vi "Main.vi"() -> ()   [LabVIEW 2018]
doc: "Use this template to build a producer/consumer design pattern with events to produce queue items. Use this design pattern instead of the User Interface Event Handler pattern for user interfaces when you want to execute code asynchronously in response to an event without slowing the user interface responsiveness."
panel:
  out "Score":i32
  in  "Grids":i32[][](array[numeric])
  in  "GridsPic":picture
  in  "stop":bool
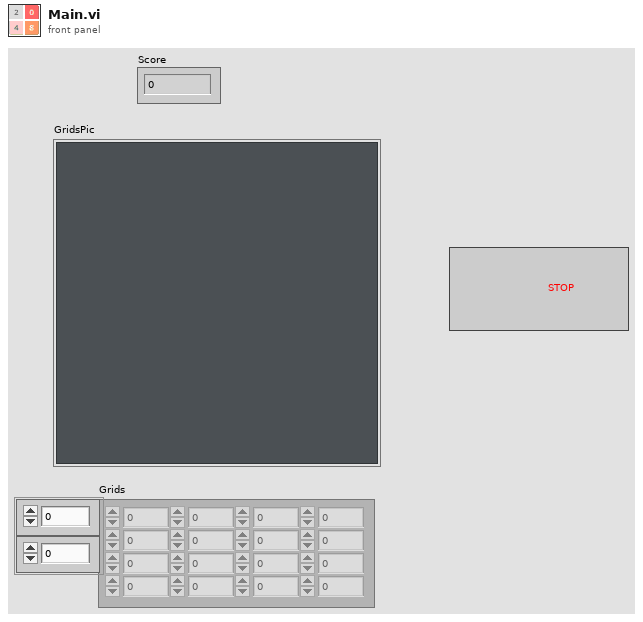
[diagram p1: front panel]
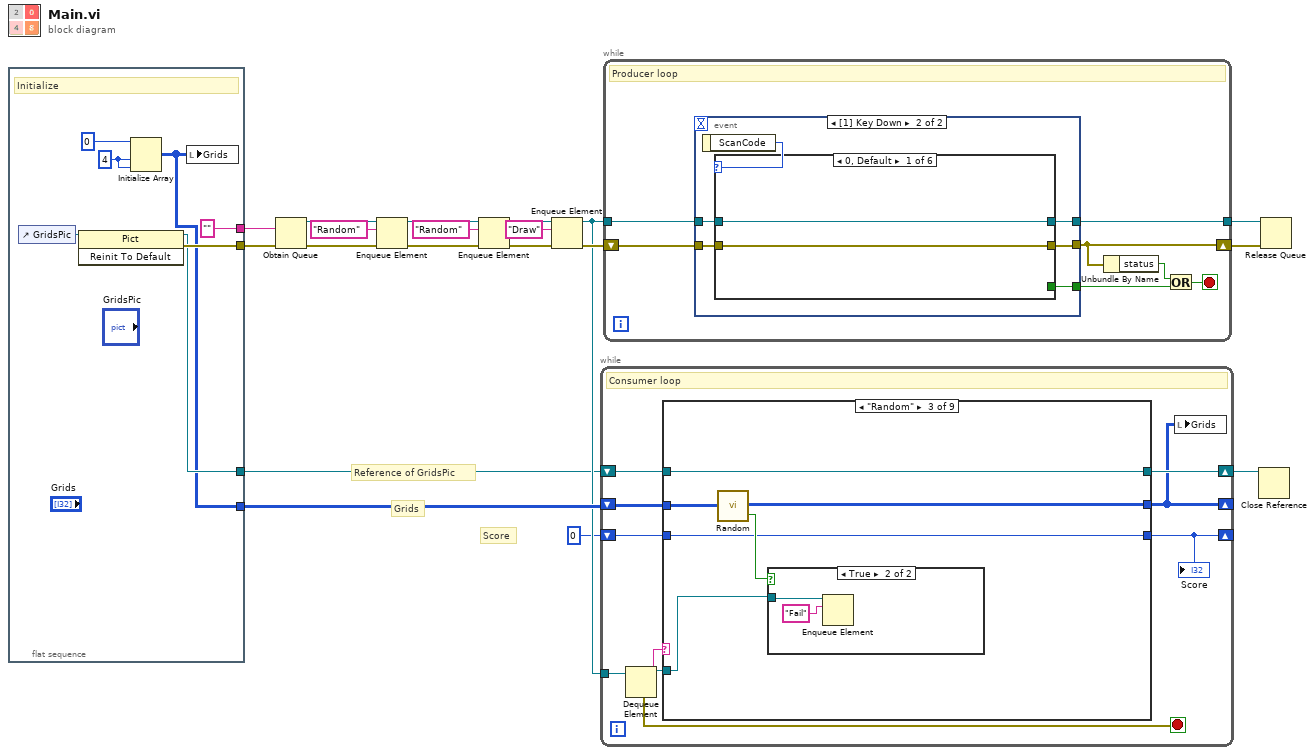
[diagram p0: block diagram]
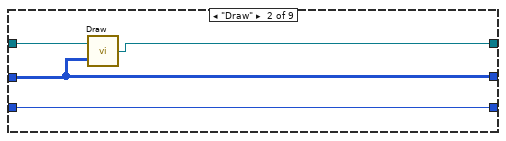
[diagram p3: hidden frame]
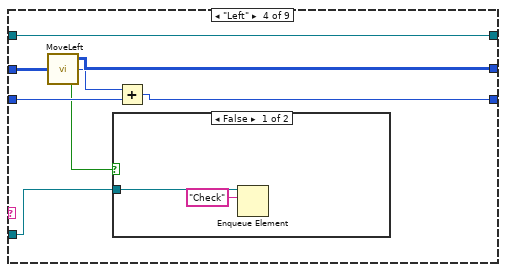
[diagram p5: hidden frame]
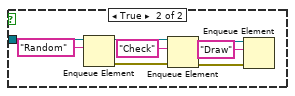
[diagram p6: hidden frame]
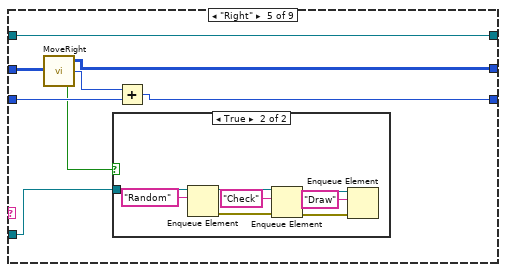
[diagram p7: hidden frame]
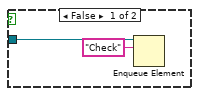
[diagram p8: hidden frame]
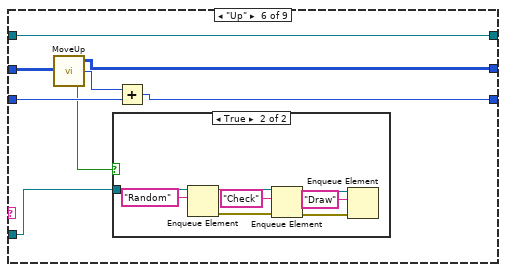
[diagram p9: hidden frame]
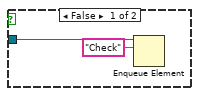
[diagram p10: hidden frame]
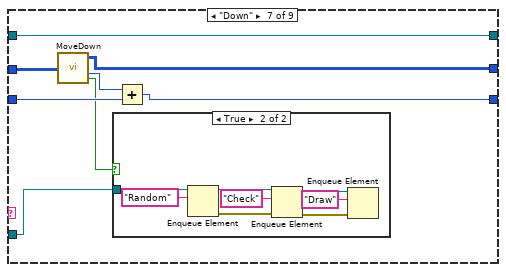
[diagram p11: hidden frame]
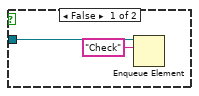
[diagram p12: hidden frame]
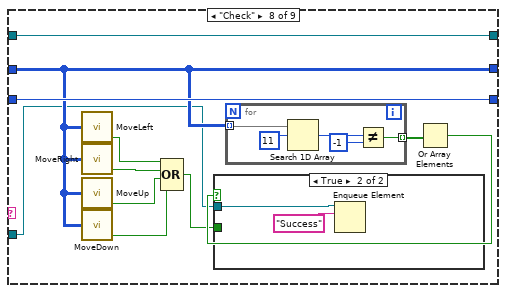
[diagram p13: hidden frame]
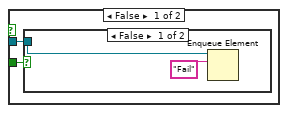
[diagram p14: hidden frame]
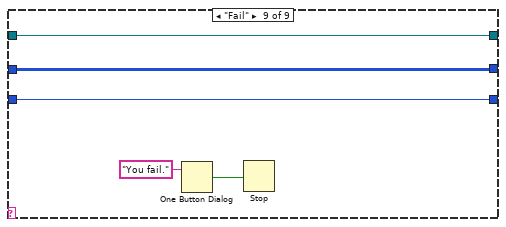
[diagram p16: hidden frame]
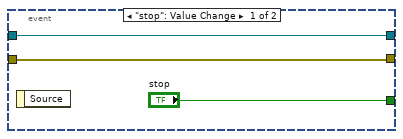
[diagram p17: hidden frame]
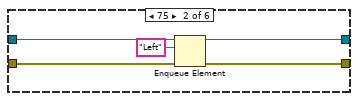
[diagram p18: hidden frame]
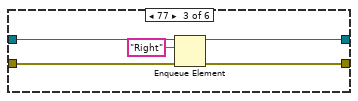
[diagram p19: hidden frame]
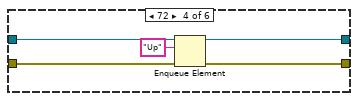
[diagram p20: hidden frame]
diagram:
  # "Score"
  # "Grids"
  # "Reference of GridsPic"
  n1 = flat-sequence {
    tunnel: [""] -> w12
    tunnel: [w19] -> w9
    tunnel: [w17] -> w7
    tunnel: [w18] -> w2
    frame #0 {
      w23 = 4 ("dimension size")
      # "Initialize"
      n2 = control-ref of="GridsPic"() -> (w20:refnum<vi>)
      n3 = invoke class="Pict" method="Reinit To Default"(reference=w20) -> (reference out=w18:refnum<vi>, error out=w19:errorcluster)  [unwired: 2 in, 1 out]
      n4 = Initialize Array(0 ("element"), w23, w23) -> (w17:i32[][])
      n5 = local write "Grids"(w17) -> ()
    }
  }
  n6 = Obtain Queue(element data type=w12, error in (no error)=w9) -> (queue out=w14:refnum<queue>, error out=w16:errorcluster)  [unwired: 3 in, 1 out]
  n7 = Enqueue Element(queue=w14, element="Random") -> (queue out=w11:refnum<queue>)  [unwired: 2 in, 2 out]
  n8 = Enqueue Element(queue=w11, element="Random") -> (queue out=w6:refnum<queue>)  [unwired: 2 in, 2 out]
  n9 = Enqueue Element(queue=w6, element="Draw") -> (queue out=w4:refnum<queue>)  [unwired: 2 in, 2 out]
  n10 = while {
    tunnel: w4 -> [w33]
    shift-right: [w29] -> w8
    shift-left: w2 -> [w31]
    shift-right: [w28] -> _
    shift-left: w7 -> [w30]
    shift-right: [w25] -> _
    shift-left: 0 ("Score") -> [w24]
    stop <- w26 stop-if-true
    # "Consumer loop"
    n11 = Dequeue Element(queue=w33) -> (queue out=w27:refnum<queue>, element=w32:string, error out=w26:errorcluster)  [unwired: 2 in, 1 out]
    n12 = case shown="\"Random\"" w32 {
      tunnel: w31 -> [w36 w40 w46 w55 w74 w92 w110 w130 w147]
      tunnel: w30 -> [w35 w39 w45 w56 w70 w88 w106 w125 w146]
      tunnel: [w36 w38 w46 w55 w74 w92 w110 w130 w147] -> w29
      tunnel: [w35 w39 w42 w54 w69 w87 w105 w125 w146] -> w28
      tunnel: w27 -> [_ _ w43 w49 w71 w89 w107 w122 _]
      tunnel: [w34 w37 w41 w51 w72 w90 w108 w131 w143] -> w25
      tunnel: w24 -> [w34 w37 w41 w52 w73 w91 w109 w131 w143]
      frame "", Default {
      }
      frame "Draw" {
        n13 = call "Draw.vi"("Grids"=w39, "Picture in"=w40) -> ("reference out"=w38:refnum<vi>)
      }
      frame "Random" {
        n14 = call "Random.vi"("Grids in"=w45) -> ("Grids out"=w42:i32[][], "Failed?"=w44:bool)
        n15 = case shown="True" w44 {
          tunnel: w43 -> [_ w48]
          frame False {
          }
          frame True {
            n16 = Enqueue Element(queue=w48, element="Fail") -> ()  [unwired: 2 in, 3 out]
          }
        }
      }
      frame "Left" {
        n17 = call "MoveLeft.vi"("Grids In"=w56) -> ("Grid Out"=w54:i32[][], "Score"=w53:i32, "Moved?"=w50:bool)
        n18 = case shown="False" w50 {
          tunnel: w49 -> [w58 w66]
          frame False {
            n19 = Enqueue Element(queue=w58, element="Check") -> ()  [unwired: 2 in, 3 out]
          }
          frame True {
            n20 = Enqueue Element(queue=w66, element="Random") -> (queue out=w63:refnum<queue>, error out=w62:errorcluster)  [unwired: 2 in, 1 out]
            n21 = Enqueue Element(queue=w63, element="Check", error in (no error)=w62) -> (queue out=w61:refnum<queue>, error out=w59:errorcluster)  [unwired: 1 in, 1 out]
            n22 = Enqueue Element(queue=w61, element="Draw", error in (no error)=w59) -> ()  [unwired: 1 in, 3 out]
          }
        }
        n23 = Add(x=w53, y=w52) -> (x+y=w51:i32)
      }
      frame "Right" {
        n24 = call "MoveRight.vi"("Grids In"=w70) -> ("Grids Out"=w69:i32[][], "Score"=w68:i32, "Moved?"=w67:bool)
        n25 = case shown="True" w67 {
          tunnel: w71 -> [w76 w84]
          frame False {
            n26 = Enqueue Element(queue=w76, element="Check") -> ()  [unwired: 2 in, 3 out]
          }
          frame True {
            n27 = Enqueue Element(queue=w84, element="Random") -> (queue out=w81:refnum<queue>, error out=w80:errorcluster)  [unwired: 2 in, 1 out]
            n28 = Enqueue Element(queue=w81, element="Check", error in (no error)=w80) -> (queue out=w79:refnum<queue>, error out=w77:errorcluster)  [unwired: 1 in, 1 out]
            n29 = Enqueue Element(queue=w79, element="Draw", error in (no error)=w77) -> ()  [unwired: 1 in, 3 out]
          }
        }
        n30 = Add(x=w68, y=w73) -> (x+y=w72:i32)
      }
      frame "Up" {
        n31 = call "MoveUp.vi"("Grids In"=w88) -> ("Grids Out"=w87:i32[][], "Score"=w86:i32, "Moved?"=w85:bool)
        n32 = case shown="True" w85 {
          tunnel: w89 -> [w94 w102]
          frame False {
            n33 = Enqueue Element(queue=w94, element="Check") -> ()  [unwired: 2 in, 3 out]
          }
          frame True {
            n34 = Enqueue Element(queue=w102, element="Random") -> (queue out=w99:refnum<queue>, error out=w98:errorcluster)  [unwired: 2 in, 1 out]
            n35 = Enqueue Element(queue=w99, element="Check", error in (no error)=w98) -> (queue out=w97:refnum<queue>, error out=w95:errorcluster)  [unwired: 1 in, 1 out]
            n36 = Enqueue Element(queue=w97, element="Draw", error in (no error)=w95) -> ()  [unwired: 1 in, 3 out]
          }
        }
        n37 = Add(x=w86, y=w91) -> (x+y=w90:i32)
      }
      frame "Down" {
        n38 = call "MoveDown.vi"("Grids In"=w106) -> ("Grids Out"=w105:i32[][], "Score"=w104:i32, "Moved?"=w103:bool)
        n39 = case shown="True" w103 {
          tunnel: w107 -> [w112 w120]
          frame False {
            n40 = Enqueue Element(queue=w112, element="Check") -> ()  [unwired: 2 in, 3 out]
          }
          frame True {
            n41 = Enqueue Element(queue=w120, element="Random") -> (queue out=w117:refnum<queue>, error out=w116:errorcluster)  [unwired: 2 in, 1 out]
            n42 = Enqueue Element(queue=w117, element="Check", error in (no error)=w116) -> (queue out=w115:refnum<queue>, error out=w113:errorcluster)  [unwired: 1 in, 1 out]
            n43 = Enqueue Element(queue=w115, element="Draw", error in (no error)=w113) -> ()  [unwired: 1 in, 3 out]
          }
        }
        n44 = Add(x=w104, y=w109) -> (x+y=w108:i32)
      }
      frame "Check" {
        n45 = call "MoveLeft.vi"("Grids In"=w125) -> ("Moved?"=w129:bool)  [unwired: 2 out]
        n46 = call "MoveRight.vi"("Grids In"=w125) -> ("Moved?"=w128:bool)  [unwired: 2 out]
        n47 = call "MoveUp.vi"("Grids In"=w125) -> ("Moved?"=w127:bool)  [unwired: 2 out]
        n48 = call "MoveDown.vi"("Grids In"=w125) -> ("Moved?"=w126:bool)  [unwired: 2 out]
        n49 = Compound Arithmetic op=OR(w129, w128, w127, w126) -> (w121:bool)
        n50 = for {
          tunnel: w125 -> [w142] mode=indexing
          tunnel: [w138] -> w124 mode=indexing
          n51 = Search 1D Array(1D array=w142, element=11) -> (index of element=w140:i32)  [unwired: 1 in]
          n52 = Not Equal?(x=w140, y=-1) -> (x != y?=w138:bool)
        }
        n53 = Or Array Elements(Boolean array=w124) -> (logical OR=w123:bool)
        n54 = case shown="True" w123 {
          tunnel: w122 -> [w132 w137]
          tunnel: w121 -> [w133 _]
          frame False {
            n55 = case shown="False" w133 {
              tunnel: w132 -> [w135 _]
              frame False {
                n56 = Enqueue Element(queue=w135, element="Fail") -> ()  [unwired: 2 in, 3 out]
              }
              frame True {
              }
            }
          }
          frame True {
            n57 = Enqueue Element(queue=w137, element="Success") -> ()  [unwired: 2 in, 3 out]
          }
        }
      }
      frame "Fail" {
        n58 = One Button Dialog(message="You fail.") -> (true=w144:bool)  [unwired: 1 in]
        n59 = Stop(stop? (T)=w144) -> ()
      }
    }
    "Score" <- w25
    n60 = local write "Grids"(w28) -> ()
  }
  n61 = while {
    shift-right: [w150] -> w15
    shift-left: w16 -> [w153]
    tunnel: w4 -> [w154]
    tunnel: [w148] -> w13
    stop <- w151 stop-if-true
    # "Producer loop"
    n62 = event shown="[1] Key Down" {
      selector: _ -> [_ _]
      dyn-events: _ -> [_ _]
      timeout: _ -> [_ _]
      tunnel: w154 -> [w155 w162]
      tunnel: w153 -> [w156 w160]
      tunnel: [w156 w159] -> w150
      tunnel: ["stop" w158] -> w152
      tunnel: [w155 w161] -> w148
      event "stop": Value Change {
        n63 = event-data() -> ()  [unwired: 1 in, 1 out]
      }
      event Key Down {
        n64 = event-data() -> ("ScanCode"=w163:i16)  [unwired: 1 in]
        n65 = case shown="0, Default" w163 {
          tunnel: w162 -> [w165 w169 w173 w177 w181 w184]
          tunnel: [w165 w166 w170 w174 w178 w184] -> w161
          tunnel: w160 -> [w164 w168 w172 w176 w180 w183]
          tunnel: [w164 w168 w172 w176 w180 w183] -> w159
          tunnel: [_ _ _ _ _ TRUE] -> w158
          frame 0, Default {
          }
          frame 75 {
            n66 = Enqueue Element(queue=w169, element="Left") -> (queue out=w166:refnum<queue>)  [unwired: 2 in, 2 out]
          }
          frame 77 {
            n67 = Enqueue Element(queue=w173, element="Right") -> (queue out=w170:refnum<queue>)  [unwired: 2 in, 2 out]
          }
          frame 72 {
            n68 = Enqueue Element(queue=w177, element="Up") -> (queue out=w174:refnum<queue>)  [unwired: 2 in, 2 out]
          }
          frame 80 {
            n69 = Enqueue Element(queue=w181, element="Down") -> (queue out=w178:refnum<queue>)  [unwired: 2 in, 2 out]
          }
          frame 1 {
            # "Esc"
          }
        }
      }
    }
    n70 = Unbundle By Name(w150) -> ("status"=w149:bool)
    n71 = Or(x=w149, y=w152) -> (x .or. y?=w151:bool)
  }
  n72 = Close Reference(reference=w8) -> ()  [unwired: 1 in, 1 out]
  n73 = Release Queue(queue=w13, error in (no error)=w15) -> ()  [unwired: 1 in, 3 out]
